vi "Get Frame Signals.vi"(6 "CAN:Frame Type":T1=enum."All", 8 "error in":errorcluster, 9 "Parent Tag":string, 10 "Tree Reference":refnum<vi>, 11 "Frms":refnum<k21>[](array[refnum])) -> (0 "error out":errorcluster, 2 "Tree Reference Out":refnum<vi>)   [LabVIEW 2015, in "Protection and Rolling Counter Addon System Explorer.lvlib"]
uses:
  Types/CAN Filter Type.ctl
  Protection and Rolling Counter Addon System Explorer.lvlib
  <resource>/objmgr/xnet.rc
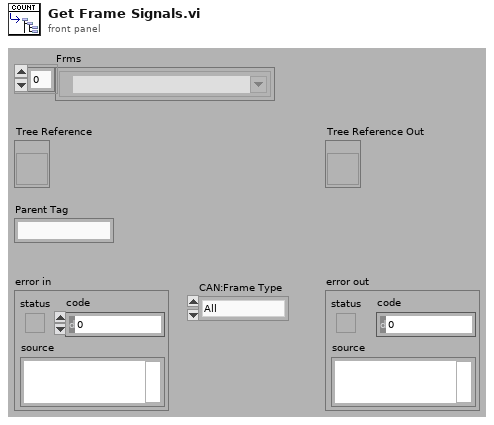
[diagram p1: front panel]
types:
  T1 = typedef "Protection and Rolling Counter Addon System Explorer.lvlib/CAN Filter Type.ctl" = enum16{"Cyclic Data", "Event Data", "Cyclic/Event", "All"}
  T2 = enum16{"open", "replace", "create", "open or create", "replace or create", "replace or create with confirmation"}
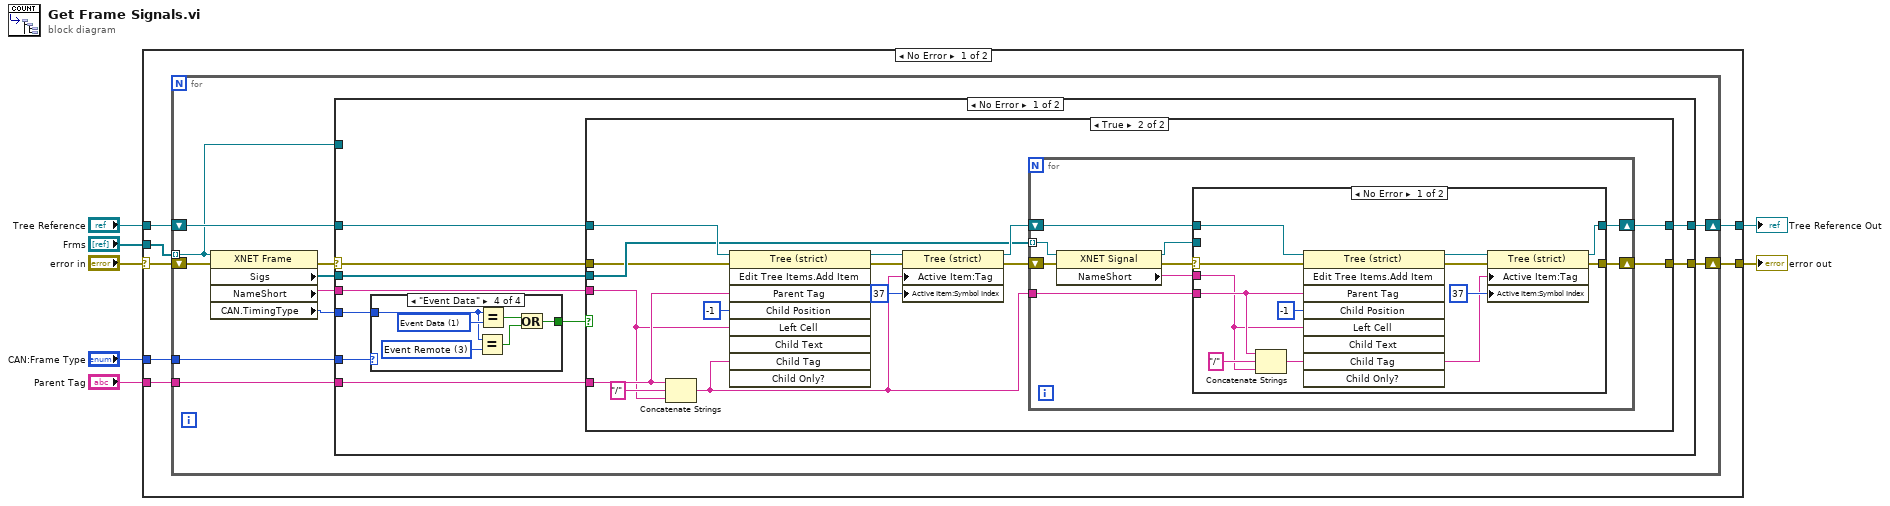
[diagram p0: block diagram]
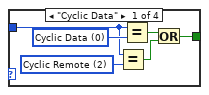
[diagram p2: hidden frame]
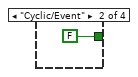
[diagram p3: hidden frame]
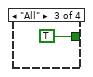
[diagram p4: hidden frame]
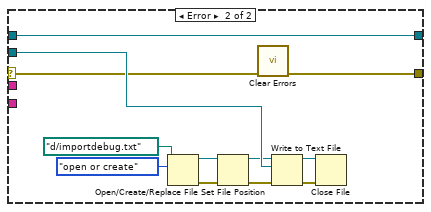
[diagram p6: hidden frame]
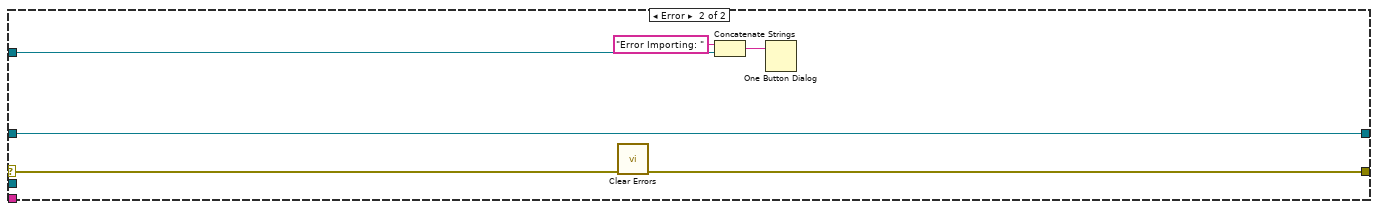
[diagram p7: hidden frame]
diagram:
  n1 = case shown="No Error" "error in" {
    selector: "error in" -> [w11 w107]
    tunnel: [w14 w107] -> w7
    tunnel: "Frms" -> [w9 _]
    tunnel: "Tree Reference" -> [w13 w106]
    tunnel: "Parent Tag" -> [w12 _]
    tunnel: [w10 w106] -> w2
    tunnel: "CAN:Frame Type" -> [w8 _]
    frame No Error {
      n2 = for {
        tunnel: w9 -> [w17] mode=indexing
        shift-right: [w20] -> w14
        shift-left: w11 -> [w25]
        tunnel: w12 -> [w23]
        shift-right: [w22] -> w10
        shift-left: w13 -> [w24]
        tunnel: w8 -> [w16]
        n3 = property class="XNET Frame"(reference=w17, error in=w25) -> (error out=w18:errorcluster, "Sigs"=w21:refnum<k21>[], "NameShort"=w19:string, "CAN.TimingType"=w15:u32)  [unwired: 1 out]
        n4 = case shown="No Error" w18 {
          selector: w18 -> [w29 w102]
          tunnel: w24 -> [w35 w100]
          tunnel: w23 -> [w34 _]
          tunnel: [w33 w100] -> w22
          tunnel: w21 -> [w32 _]
          tunnel: [w31 w101] -> w20
          tunnel: w19 -> [w30 _]
          tunnel: w17 -> [_ w105]
          tunnel: w16 -> [w26 _]
          tunnel: w15 -> [w28 _]
          frame No Error {
            n5 = case shown="\"Event Data\"" w26 {
              tunnel: w28 -> [w38 _ _ w47]
              tunnel: [w36 FALSE TRUE w45] -> w27
              frame "Cyclic Data" {
                w40 = u32 2 items=["Cyclic Data", "Event Data", "Cyclic Remote", "Event Remote", "Cyclic/Event"] ("CAN:Timing Type")
                w41 = u32 0 items=["Cyclic Data", "Event Data", "Cyclic Remote", "Event Remote", "Cyclic/Event"] ("CAN:Timing Type")
                n6 = Equal?(x=w38, y=w40) -> (x = y?=w39:bool)
                n7 = Equal?(x=w38, y=w41) -> (x = y?=w37:bool)
                n8 = Or(x=w37, y=w39) -> (x .or. y?=w36:bool)
              }
              frame "Cyclic/Event" {
              }
              frame "All" {
              }
              frame "Event Data" {
                w46 = u32 3 items=["Cyclic Data", "Event Data", "Cyclic Remote", "Event Remote", "Cyclic/Event"] ("CAN:Timing Type")
                w48 = u32 1 items=["Cyclic Data", "Event Data", "Cyclic Remote", "Event Remote", "Cyclic/Event"] ("CAN:Timing Type")
                n9 = Equal?(x=w47, y=w46) -> (x = y?=w44:bool)
                n10 = Equal?(x=w47, y=w48) -> (x = y?=w49:bool)
                n11 = Or(x=w49, y=w44) -> (x .or. y?=w45:bool)
              }
            }
            n12 = case shown="True" w27 {
              tunnel: w35 -> [w51 w66]
              tunnel: w34 -> [_ w63]
              tunnel: [w51 w62] -> w33
              tunnel: w32 -> [_ w55]
              tunnel: [w50 w54] -> w31
              tunnel: w30 -> [_ w53]
              tunnel: w29 -> [w50 w52]
              frame False {
              }
              frame True {
                n13 = Concatenate Strings(w63, "/" ("string"), w53) -> (w56:string)
                n14 = invoke on="Invoke Node" class="Tree (strict)" method="Edit Tree Items.Add Item"(reference=w66, error in=w52, "Parent Tag"=w63, "Child Position"=-1, "Left Cell"=w53, "Child Tag"=w56) -> (reference out=w59:refnum<vi>, error out=w60:errorcluster)  [unwired: 3 in, 7 out]
                n15 = property class="Tree (strict)"(reference=w59, error in=w60, "Active Item:Tag"=w56, "Active Item:Symbol Index"=37) -> (reference out=w57:refnum<vi>, error out=w58:errorcluster)
                n16 = for {
                  tunnel: w55 -> [w68] mode=indexing
                  shift-right: [w70] -> w54
                  shift-left: w58 -> [w75]
                  tunnel: w56 -> [w73]
                  shift-right: [w71] -> w62
                  shift-left: w57 -> [w74]
                  n17 = property class="XNET Signal"(reference=w68, error in=w75) -> (reference out=w67:refnum<k21>, error out=w69:errorcluster, "NameShort"=w72:string)
                  n18 = case shown="No Error" w69 {
                    selector: w69 -> [w76 w97]
                    tunnel: w74 -> [w87 w99]
                    tunnel: w73 -> [w85 _]
                    tunnel: w72 -> [w84 _]
                    tunnel: [w79 w99] -> w71
                    tunnel: [w77 w96] -> w70
                    tunnel: w67 -> [_ w98]
                    frame No Error {
                      n19 = Concatenate Strings(w85, "/" ("string"), w84) -> (w78:string)
                      n20 = invoke on="Invoke Node" class="Tree (strict)" method="Edit Tree Items.Add Item"(reference=w87, error in=w76, "Parent Tag"=w85, "Child Position"=-1, "Left Cell"=w84, "Child Tag"=w78) -> (reference out=w80:refnum<vi>, error out=w81:errorcluster)  [unwired: 3 in, 7 out]
                      n21 = property class="Tree (strict)"(reference=w80, error in=w81, "Active Item:Tag"=w78, "Active Item:Symbol Index"=37) -> (reference out=w79:refnum<vi>, error out=w77:errorcluster)
                    }
                    frame Error {
                      n22 = Open/Create/Replace File(file path (use dialog)=path "d:/importdebug.txt", operation (0:open)=T2."open or create") -> (refnum out=w93:refnum<file>, error out=w94:errorcluster)  [unwired: 4 in, 1 out]
                      n23 = Set File Position(refnum=w93, error in=w94) -> (refnum out=w92:refnum<file>, error out=w91:errorcluster)  [unwired: 2 in]
                      n24 = call <vilib>:"Clear Errors.vi"("error in (no error)"=w97) -> ("error out"=w96:errorcluster)  [unwired: 5 in, 1 out]
                      n25 = Write to Text File(file (use dialog)=w92, text=w98, error in=w91) -> (refnum out=w89:refnum<file>, error out=w90:errorcluster)  [unwired: 1 in, 1 out]
                      n26 = Close File(refnum=w89, error in=w90) -> ()  [unwired: 2 out]
                    }
                  }
                }
              }
            }
          }
          frame Error {
            n27 = call <vilib>:"Clear Errors.vi"("error in (no error)"=w102) -> ("error out"=w101:errorcluster)  [unwired: 5 in, 1 out]
            n28 = Concatenate Strings("Error Importing: " ("string"), w105) -> (w103:string)
            n29 = One Button Dialog(message=w103) -> ()  [unwired: 1 in, 1 out]
          }
        }
      }
    }
    frame Error {
    }
  }
  "error out" <- w7
  "Tree Reference Out" <- w2
